vi "To And From String Array Test.vi"() -> ()   [LabVIEW 2015, in "String Compare Tests.lvlib"]
uses:
  String Compare Tests.lvlib
  Config/String Compare Config.lvclass
  <vilib>/NI/Tag Bus/tag/Data Type.ctl
  <vilib>/NI/Tag Bus Module Framework/channel/channel classification.ctl
  Config/Mode.ctl
  Config/String Compare Config.lvclass/String Compare Config.ctl
  Config/Write Test Value Channel.vi
  Config/Write Result Channel.vi
  Config/Write Mode.vi
  Config/Write Limit_Regex.vi
  Config/Write ignore case.vi
  Config/Write Multiline.vi
  Config/Write Offset.vi
  <vilib>/NI/Tag Bus/tag/tag descriptor.lvclass
  <vilib>/NI/Tag Bus Module Framework/channel/TBM channel.lvclass
panel:
  out "error out":errorcluster
  out "Pass":bool
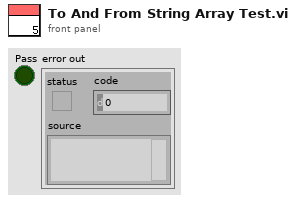
[diagram p1: front panel]
types:
  T1 = typedef "Mode.ctl" = enum16{"Compare Strings", "Match Regex"}
  T2 = typedef "TBM channel.lvclass/channel classification.ctl" = enum16{"input data", "output data", "processing parameter", "processing result"}
  T3 = typedef "tag bus.lvlib/tag descriptor.lvclass/Data Type.ctl" = enum16{"Double", "Single", "I64", "I32", "I16", "I8", "U64", "U32", "U16", "U8", "Boolean", "String", "Array of Double", "Array of Single", "Array of I64", "Array of I32", "Array of I16", "Array of I8", "Array of U64", "Array of U32", "Array of U16", "Array of U8", "Array of Boolean", "Array of String"}
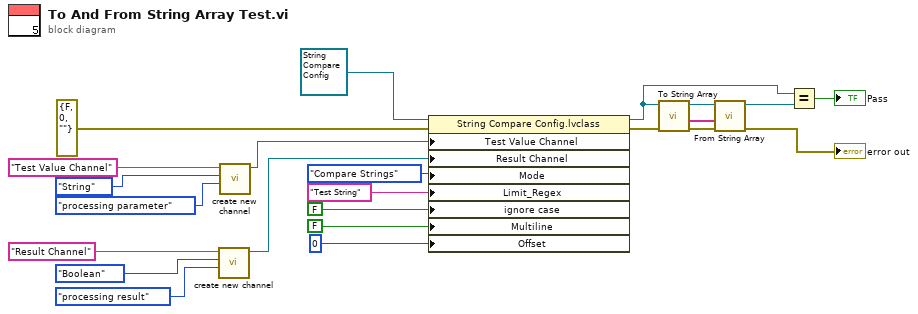
[diagram p0: block diagram]
diagram:
  n1 = call <vilib>:"create new channel.vi"("channel classification"=channel_classification."processing result", "data type"=Data_Type."Boolean", "channel name"="Result Channel") -> ("channel"=w10:refnum<class "TBM channel.lvclass">)  [unwired: 8 in]
  n2 = call <vilib>:"create new channel.vi"("channel classification"=channel_classification."processing parameter", "data type"=Data_Type."String" ("Data Type"), "channel name"="Test Value Channel" ("Jump Tag Name")) -> ("channel"=w14:refnum<class "TBM channel.lvclass">)  [unwired: 8 in]
  n3 = property class="String Compare Config.lvclass"(reference=refnum<class "String Compare Config.lvclass"> refnum ("String Compare Config.lvclass"), error in=errorcluster {"status"=FALSE, "code"=0, "source"=""} ("error in (no error)"), "Test Value Channel"=w14, "Result Channel"=w10, "Mode"=Mode."Compare Strings", "Limit_Regex"="Test String", "ignore case"=FALSE, "Multiline"=FALSE, "Offset"=0) -> (reference out=w2:refnum<class "String Compare Config.lvclass">, error out=w20:errorcluster)
  n4 = call-dynamic "To String Array.vi"("error in (no error)"=w20, "String Compare Config in"=w2) -> ("error out"=w19:errorcluster, "Step String Array"=w3:string[], "String Compare Config out"=w22:refnum<class "String Compare Config.lvclass">)  [unwired: 7 in]
  n5 = call-dynamic "From String Array.vi"("error in (no error)"=w19, "String Array"=w3, "String Compare Config in"=w22) -> ("error out"=→"error out":errorcluster, "String Compare Config out"=w1:refnum<class "String Compare Config.lvclass">)  [unwired: 5 in, 2 out]
  n6 = Equal?(x=w2, y=w1) -> (x = y?=→"Pass":bool)
